vi "Read State.vi"(8 "error in (no error)":errorcluster, 10 "Shutter-NP":T1, 11 "Container in":refnum<class "Container.lvclass">) -> (0 "error out":errorcluster, 2 "Shutter-NP out":T1, 3 "Container out":refnum<class "Container.lvclass">)   [LabVIEW 2016, in "Container.lvclass"]
uses:
  Container.lvclass
  Controls/Shutters.ctl
  Controls/Shutter Data.ctl
  Controls/Shutter States.ctl
  Container.lvclass/Container.ctl
  Sci/SciShutt.lvclass
  LFCSim/LFCSimShutt.lvclass
  ExtFlat/ExtFlatShutt.lvclass
  SimFlat/SimFlatShutt.lvclass
  Solar/SolarShutt.lvclass
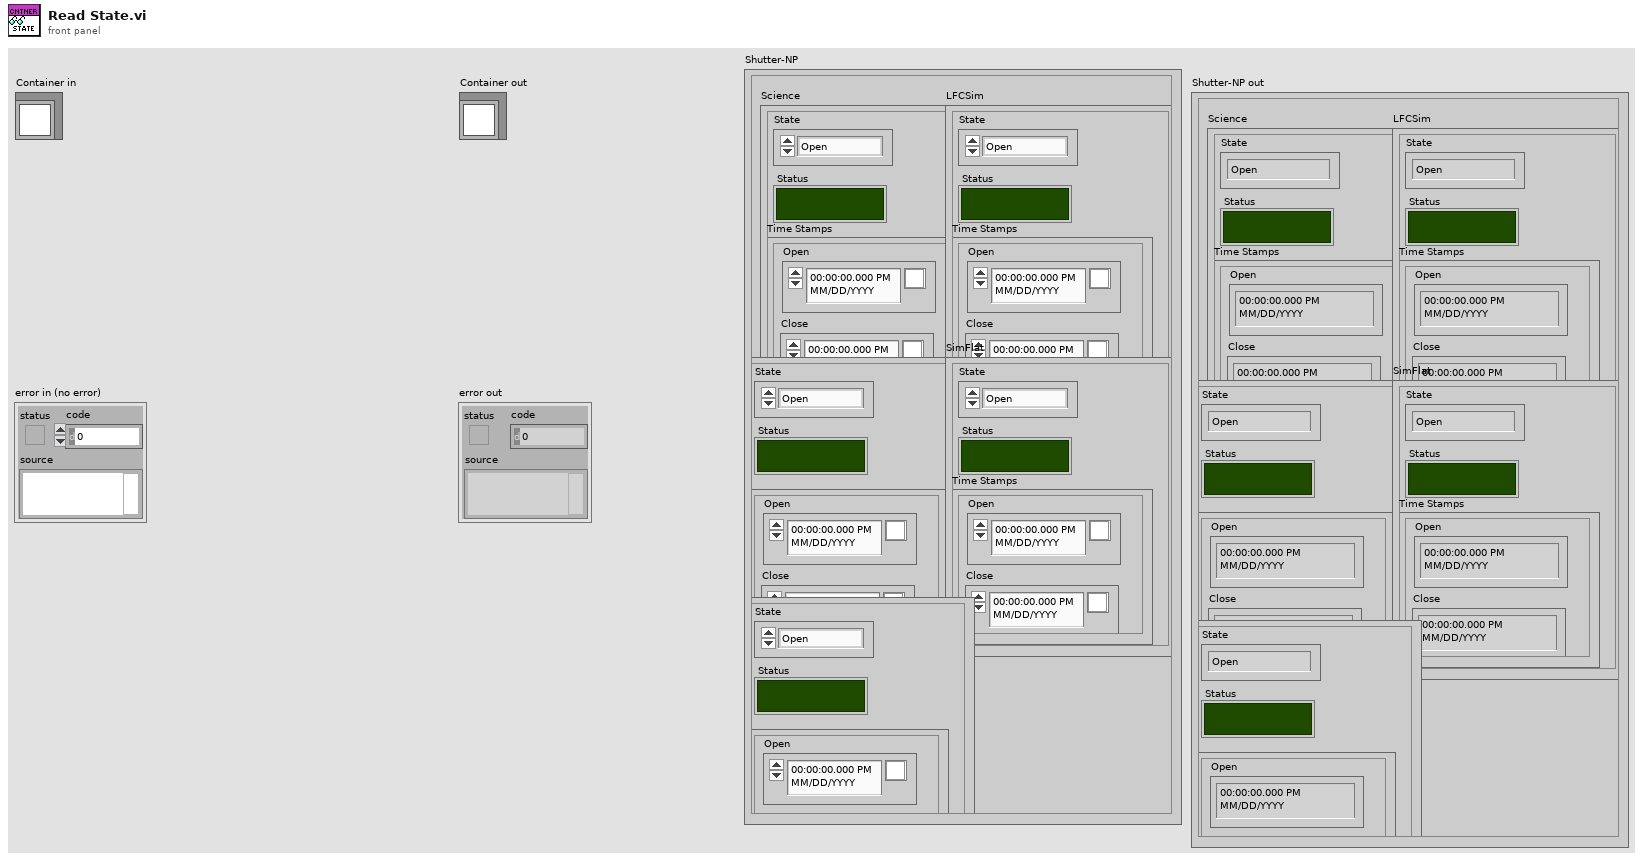
[diagram p1: front panel]
types:
  T1 = typedef "Shutters.ctl" = cluster{"Science":T2, "LFCSim":T2, "ExtendFlat":T2, "SimFlat":T2, "Solar":T2}
  T2 = typedef "Shutter Data.ctl" = cluster{"Status":bool, "State":T3, "Time Stamps":cluster{"Open":timestamp, "Close":timestamp}}
  T3 = typedef "Shutter States.ctl" = enum16{"Open", "Close", "Wait", "Off", "Arm", "Idle"}
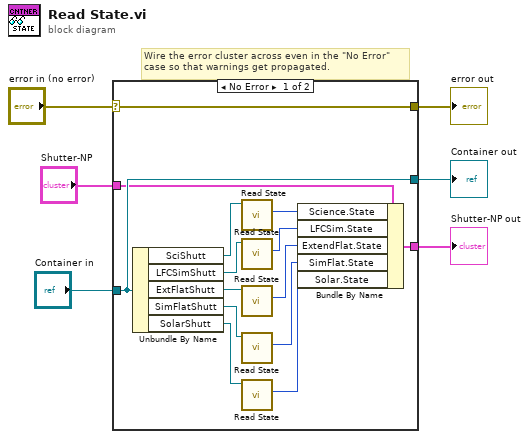
[diagram p0: block diagram]
diagram:
  # "Wire the error cluster across even in the \"No Error\"\ncase so that warnings get propagated."
  n1 = case shown="No Error" "error in (no error)" {
    selector: "error in (no error)" -> [w20 w23]
    tunnel: [w20 w23] -> w5
    tunnel: [w15 w22] -> w3
    tunnel: "Container in" -> [w15 w22]
    tunnel: "Shutter-NP" -> [w13 w21]
    tunnel: [w12 w21] -> w1
    frame No Error {
      n2 = Unbundle By Name(w15) -> ("SciShutt"=w19:refnum<class "SciShutt.lvclass">, "LFCSimShutt"=w18:refnum<class "LFCSimShutt.lvclass">, "ExtFlatShutt"=w14:refnum<class "ExtFlatShutt.lvclass">, "SimFlatShutt"=w17:refnum<class "SimFlatShutt.lvclass">, "SolarShutt"=w16:refnum<class "SolarShutt.lvclass">)
      n3 = call-dynamic "Read State.vi"("Shutter in"=w19) -> ("State"=w11:T3)  [unwired: 8 in, 2 out]
      n4 = call-dynamic "Read State.vi"("Shutter in"=w18) -> ("State"=w10:T3)  [unwired: 8 in, 2 out]
      n5 = call-dynamic "Read State.vi"("Shutter in"=w14) -> ("State"=w9:T3)  [unwired: 8 in, 2 out]
      n6 = call-dynamic "Read State.vi"("Shutter in"=w17) -> ("State"=w8:T3)  [unwired: 8 in, 2 out]
      n7 = call-dynamic "Read State.vi"("Shutter in"=w16) -> ("State"=w7:T3)  [unwired: 8 in, 2 out]
      n8 = Bundle By Name(cluster=w13, "Science.State"=w11, "LFCSim.State"=w10, "ExtendFlat.State"=w9, "SimFlat.State"=w8, "Solar.State"=w7) -> (w12:T1)
    }
    frame Error {
    }
  }
  "error out" <- w5
  "Container out" <- w3
  "Shutter-NP out" <- w1
